vi "Example DS18b20 Read.vi"() -> ()   [LabVIEW 2014]
uses:
  vi.lib/Q-WaveSystems/QwaveSys Raspberry Pi for LabVIEW Home-Education/QwaveSys Raspberry Pi Library.lvlib
panel:
  in  "id":string="28-000006ca18d4"
  out "standard output":string
  in  "Read Temp (T),Read ID (F)":bool
  out "Temp":dbl
  # "s"
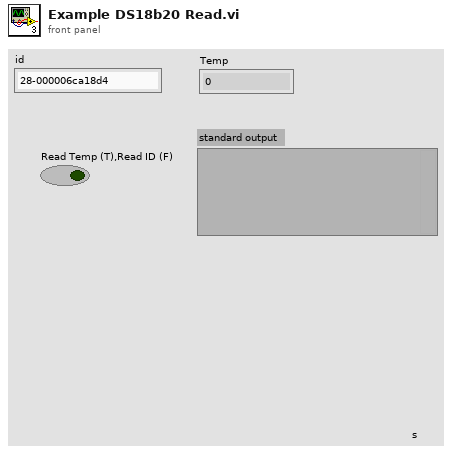
[diagram p1: front panel]
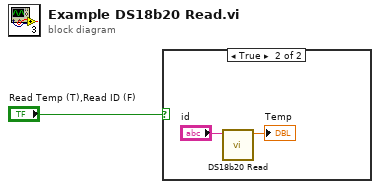
[diagram p0: block diagram]
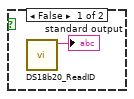
[diagram p2: hidden frame]
diagram:
  n1 = case shown="True" "Read Temp (T),Read ID (F)" {
    frame False {
      n2 = call "DS18b20_ReadID.vi"() -> ("standard output"=→"standard output":string)  [unwired: 10 in, 1 out]
    }
    frame True {
      n3 = call "DS18b20 Read.vi"("id"="id") -> ("Temp"=→"Temp":dbl)  [unwired: 9 in, 1 out]
    }
  }
